vi "Create AI Tasks.vi"(8 "error in":errorcluster, 11 "DAQmx in":refnum<class "DAQmx.lvclass">) -> (0 "error out":errorcluster, 3 "DAQmx out":refnum<class "DAQmx.lvclass">)   [LabVIEW 2019, in "DAQmx.lvclass"]
uses:
  DAQmx.lvclass
  DAQmx.lvclass/DAQmx.ctl
  <vilib>/DAQmx/create/channels.llb/DAQmx Create Channel (AI-Voltage-Basic).vi
  <resource>/objmgr/daqmx.rc
panel:
  out "Array":T1(array[cluster])
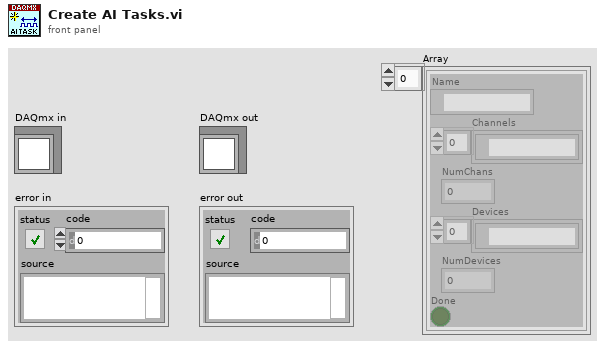
[diagram p1: front panel]
types:
  T1 = cluster{"Name":refnum<k21>, "Channels":refnum<k21>[], "NumChans":u32, "Devices":tag[], "NumDevices":u32, "Done":bool}[]
  T2 = typedef "DAQmx.lvclass/DAQ.Config.AI--Cluster--Array.ctl" = T3[]
  T3 = typedef "DAQmx.lvclass/DAQ.Config.AI--Cluster.ctl" = cluster{"Channels":tag, "Coupling":T4, "Range":T5, "input terminal configuration":i32, "Type":T6}
  T4 = typedef "DAQmx.lvclass/DAQ.Config.AI.Coupling--enum.ctl" = u16
  T5 = typedef "DAQmx.lvclass/DAQ.Config.AI.Range--enum.ctl" = enum16{"±0.316", "±1.00", "±3.16", "±10.0", "±31.6", "±42.4", ""}
  T6 = typedef "DAQmx.lvclass/DAQ.Config.Device Type--enum.ctl" = enum16{"None", "USB-4431", "PXI-446x"}
  T7 = cluster{"Name":refnum<k21>, "Channels":refnum<k21>[], "NumChans":u32, "Devices":tag[], "NumDevices":u32, "Done":bool}
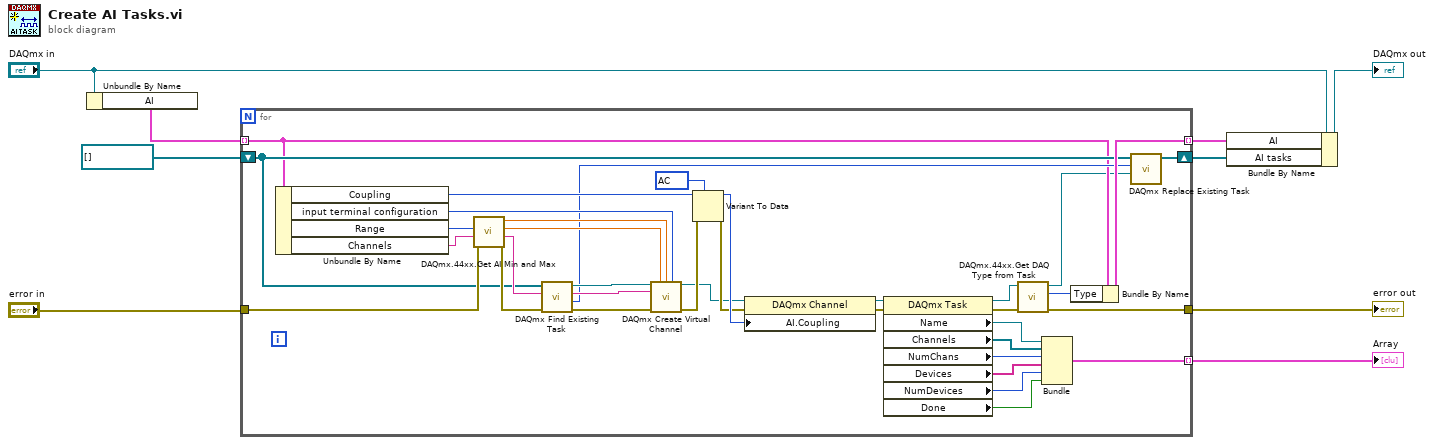
[diagram p0: block diagram]
diagram:
  n1 = Unbundle By Name("DAQmx in") -> ("AI"=w4:T2)
  n2 = for {
    tunnel: [w45] -> w7 mode=indexing
    tunnel: w4 -> [w16] mode=indexing
    tunnel: "error in" -> [w44]
    tunnel: [w10] -> w1
    tunnel: [w43] -> w3 mode=indexing
    shift-right: [w24] -> w5
    shift-left: refnum<k21>[] [] -> [w18]
    w36 = 10045 items=["AC"=10045, "DC"=10050, "GND"=10066] ("AI.Coupling")
    n3 = Unbundle By Name(w16) -> ("Coupling"=w38:T4, "input terminal configuration"=w42:i32, "Range"=w39:T5, "Channels"=w25:tag)
    n4 = call "DAQmx.44xx.Get AI Min and Max.vi"("error in (no error)"=w44, "AI.channels"=w25, "AI.Range"=w39) -> ("error out"=w23:errorcluster, "AI.channels out"=w21:tag, "AI.Max"=w40:dbl, "AI.Min"=w41:dbl)  [unwired: 5 in]
    n5 = call "DAQmx Find Existing Task.vi"("error in (no error)"=w23, "Channels"=w21, "Tasks in"=w18) -> ("error out"=w22:errorcluster, "Task Index"=w17:i32, "Channel out"=w20:tag, "Task out"=w19:refnum<k21>)  [unwired: 5 in]
    n6 = call-poly <vilib>:"DAQmx Create Virtual Channel.vi"("task in"=w19, "maximum value"=w40, "minimum value"=w41, "input terminal configuration"=w42, "physical channels"=w20, "error in"=w22) -> ("task out"=w26:refnum<k21>, "error out"=w34:errorcluster)  [unwired: 8 in]
    n7 = Variant To Data(error in=w34, type=w36, Variant=w38) -> (data=w35:i32, error out=w33:errorcluster)
    n8 = property class="DAQmx Channel"(reference=w26, error in=w33, "AI.Coupling"=w35) -> (reference out=w14:refnum<k21>, error out=w15:errorcluster)
    n9 = property class="DAQmx Task"(reference=w14, error in=w15) -> (reference out=w12:refnum<k21>, error out=w13:errorcluster, "Name"=w28:refnum<k21>, "Channels"=w27:refnum<k21>[], "NumChans"=w32:u32, "Devices"=w29:tag[], "NumDevices"=w30:u32, "Done"=w31:bool)
    n10 = call "DAQmx.44xx.Get DAQ Type from Task.vi"("error in (no error)"=w13, "Task in"=w12) -> ("error out"=w10:errorcluster, "DAQ Type"=w37:T6, "Task out"=w11:refnum<k21>)  [unwired: 6 in, 1 out]
    n11 = Bundle("Name"=w28, "Channels"=w27, "NumChans"=w32, "Devices"=w29, "NumDevices"=w30, "Done"=w31) -> (w43:T7)  [unwired: 1 in]
    n12 = Bundle By Name(cluster=w16, "Type"=w37) -> (w45:T3)
    n13 = call "DAQmx Replace Existing Task.vi"("Task in"=w11, "Task Index"=w17, "Tasks in"=w18) -> ("Tasks out"=w24:refnum<k21>[])  [unwired: 8 in]
  }
  "error out" <- w1
  "Array" <- w3
  n14 = Bundle By Name(cluster="DAQmx in", "AI"=w7, "AI tasks"=w5) -> (→"DAQmx out":refnum<class "DAQmx.lvclass">)
